vi "Write Job.vi"(10 "Job.lvclass":refnum<class "Job.lvclass">, 11 "Jobber Proxy in":refnum<class "Jobber Proxy.lvclass">) -> (3 "Jobber Proxy out":refnum<class "Jobber Proxy.lvclass">)   [LabVIEW 2014, in "Jobber Proxy.lvlib" / "Jobber Proxy.lvclass"]
uses:
  Jobber Proxy.lvclass
  Classes/Job/Job.lvclass
  Jobber Proxy.lvclass/Jobber Proxy.ctl
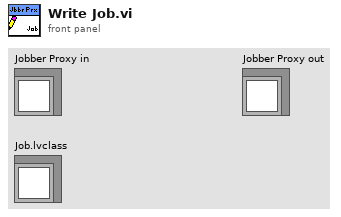
[diagram p1: front panel]
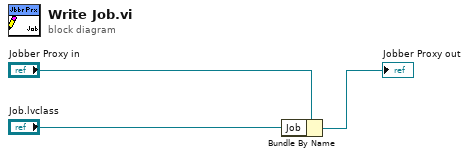
[diagram p0: block diagram]
diagram:
  n1 = Bundle By Name(cluster="Jobber Proxy in", "Job"="Job.lvclass") -> (→"Jobber Proxy out":refnum<class "Jobber Proxy.lvclass">)
